vi "Facade Line Chart.vi"(0 "Data In":T4, 2 "Display State In":T2, 3 "Container State":T3) -> (6 "Data Out":T4, 7 "Display State Out":T2, 8 "Action":T1)   [LabVIEW 2016, in "Line Chart.xctl"]
uses:
  Line Chart.xctl
  Data Line Chart.ctl
  <vilib>/_xctls/Container State.ctl
  State Line Chart.ctl
  <vilib>/_xctls/Action.ctl
  <vilib>/_xctls/XControlSupport.lvlib
panel:
  in  "ActiveX Container":refnum<k7>(container)
types:
  T1 = typedef "XControlSupport.lvlib/Action.ctl" = cluster{"Data Changed?":bool, "State Changed?":bool, "Action Name":string}
  T2 = typedef "Line Chart.xctl/State Line Chart.ctl" = cluster{"Numeric":dbl}
  T3 = typedef "XControlSupport.lvlib/Container State.ctl" = cluster{"Indicator?":bool, "Run Mode?":bool, " Refnum":refnum<vi>}
  T4 = typedef "Line Chart.xctl/Data Line Chart.ctl" = cluster{"X-Axis":string[], "Plots":cluster{"Data":dbl[], "Label":string, "Y-Axis":enum16{"Y-Axis 1", "Y-Axis 2"}, "Color":u32}[], "Plot Title":string}
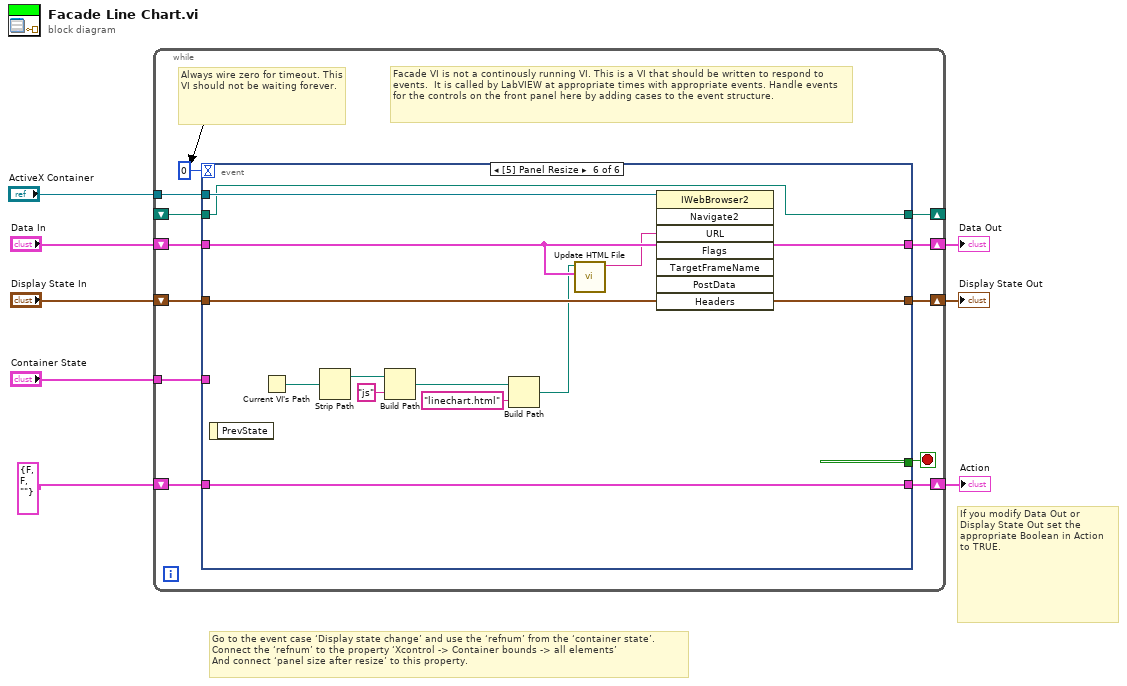
[diagram p0: block diagram]
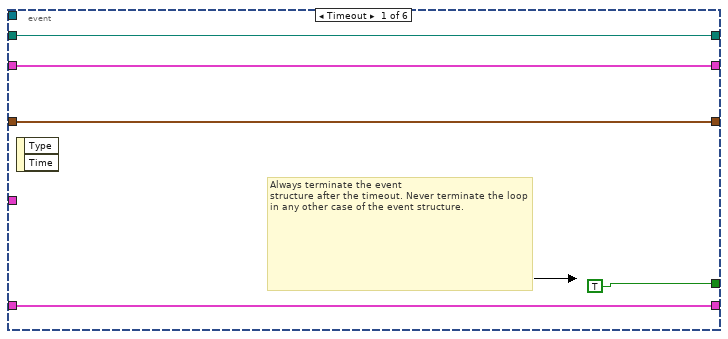
[diagram p2: hidden frame]
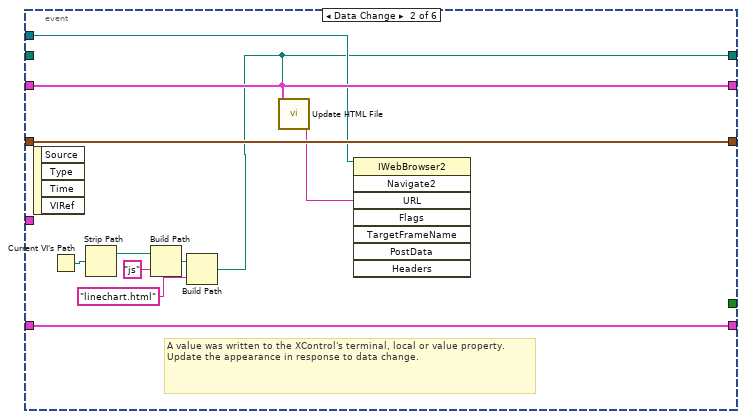
[diagram p3: hidden frame]
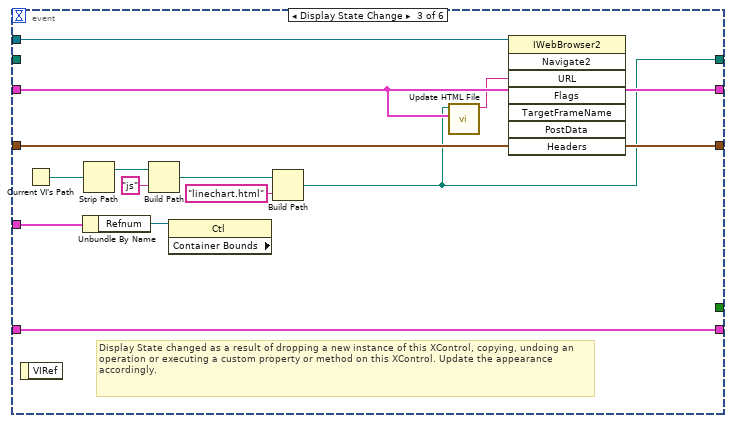
[diagram p4: hidden frame]
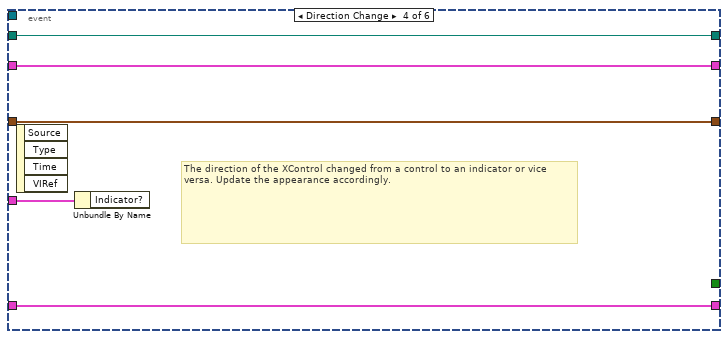
[diagram p5: hidden frame]
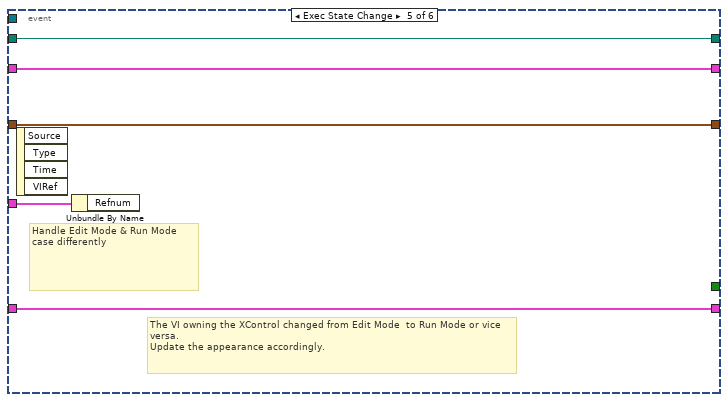
[diagram p6: hidden frame]
diagram:
  # "Go to the event case ‘Display state change’ and use the ‘refnum’ from the ‘container state’.\nConnect the ‘refnum’ to the property ‘Xcontrol -> Container bounds -> all elements’\nAnd connect ‘panel size after resize’ to this property."
  # "If you modify Data Out or\nDisplay State Out set the\nappropriate Boolean in Action\nto TRUE."
  n1 = while {
    shift-right: [w19] -> w5
    shift-left: "Display State In" -> [w20]
    tunnel: "Container State" -> [w16]
    shift-right: [w14] -> w8
    shift-left: "Data In" -> [w15]
    shift-right: [w12] -> w3
    shift-left: T1 {"Data Changed?"=FALSE, "State Changed?"=FALSE, "Action Name"=""} ("Action") -> [w13]
    tunnel: "ActiveX Container" -> [w11]
    shift-right: [w10] -> _
    shift-left: _ -> [w9]
    stop <- w18 stop-if-true
    # "Facade VI is not a continously running VI. This is a VI that should be written to respond to events.  It is called by LabVIEW at appropriate times with appropriate events. Handle events for the controls on the front panel here by adding cases to the event structure."
    # "Always wire zero for timeout. This\nVI should not be waiting forever."
    n2 = event shown="[5] Panel Resize" {
      selector: _ -> [_ _ _ _ _ _]
      dyn-events: _ -> [_ _ _ _ _ _]
      timeout: 0 -> [_ _ _ _ _ _]
      tunnel: w20 -> [w23 w36 w49 w53 w58 w71]
      tunnel: [w23 w36 w49 w53 w58 w71] -> w19
      tunnel: [TRUE _ _ _ _ _] -> w18
      tunnel: w16 -> [_ _ w47 w54 w59 _]
      tunnel: w15 -> [w22 w34 w39 w52 w57 w68]
      tunnel: [w22 w34 w39 w52 w57 w68] -> w14
      tunnel: [w24 w35 w48 w51 w56 w70] -> w12
      tunnel: w13 -> [w24 w35 w48 w51 w56 w70]
      tunnel: w11 -> [_ w33 w41 _ _ w69]
      tunnel: [w21 w31 w38 w50 w55 w67] -> w10
      tunnel: w9 -> [w21 _ _ w50 w55 w67]
      event Timeout {
        # "Always terminate the event\nstructure after the timeout. Never terminate the loop in any other case of the event structure."
        n3 = event-data() -> ()  [unwired: 1 in, 2 out]
      }
      event Data Change {
        # "A value was written to the XControl's terminal, local or value property.\nUpdate the appearance in response to data change."
        n4 = event-data() -> ()  [unwired: 1 in, 4 out]
        n5 = Current VI's Path() -> (path=w30:path)
        n6 = Strip Path(path=w30) -> (stripped path=w29:path)  [unwired: 1 out]
        n7 = Build Path(base path=w29, name or relative path="js") -> (appended path=w27:path)
        n8 = Build Path(base path=w27, name or relative path="linechart.html") -> (appended path=w31:path)
        n9 = call "Update HTML File.vi"("Data In"=w34, "Path"=w31) -> ("URL out"=w32:string)  [unwired: 9 in]
        n10 = invoke class="IWebBrowser2" method="Navigate2"(reference=w33, "URL"=w32) -> ()  [unwired: 6 in, 8 out]
      }
      event Display State Change {
        # "Display State changed as a result of dropping a new instance of this XControl, copying, undoing an operation or executing a custom property or method on this XControl. Update the appearance accordingly."
        n11 = event-data() -> ()  [unwired: 1 in, 1 out]
        n12 = Current VI's Path() -> (path=w46:path)
        n13 = Unbundle By Name(w47) -> ("Refnum"=w40:refnum<vi>)
        n14 = Strip Path(path=w46) -> (stripped path=w45:path)  [unwired: 1 out]
        n15 = Build Path(base path=w45, name or relative path="js") -> (appended path=w43:path)
        n16 = property class="Ctl" props=["Container Bounds"](reference=w40) -> ()  [unwired: 1 in, 3 out]
        n17 = Build Path(base path=w43, name or relative path="linechart.html") -> (appended path=w38:path)
        n18 = call "Update HTML File.vi"("Data In"=w39, "Path"=w38) -> ("URL out"=w37:string)  [unwired: 9 in]
        n19 = invoke class="IWebBrowser2" method="Navigate2"(reference=w41, "URL"=w37) -> ()  [unwired: 6 in, 8 out]
      }
      event Direction Change {
        # "The direction of the XControl changed from a control to an indicator or vice versa. Update the appearance accordingly."
        n20 = event-data() -> ()  [unwired: 1 in, 4 out]
        n21 = Unbundle By Name(w54) -> ()  [unwired: 1 out]
      }
      event Exec State Change {
        # "The VI owning the XControl changed from Edit Mode  to Run Mode or vice versa.\nUpdate the appearance accordingly."
        # "Handle Edit Mode & Run Mode\ncase differently"
        n22 = event-data() -> ()  [unwired: 1 in, 4 out]
        n23 = Unbundle By Name(w59) -> ()  [unwired: 1 out]
      }
      event Panel Resize {
        n24 = event-data() -> ()  [unwired: 1 in, 1 out]
        n25 = Current VI's Path() -> (path=w65:path)
        n26 = Strip Path(path=w65) -> (stripped path=w64:path)  [unwired: 1 out]
        n27 = Build Path(base path=w64, name or relative path="js") -> (appended path=w62:path)
        n28 = Build Path(base path=w62, name or relative path="linechart.html") -> (appended path=w60:path)
        n29 = call "Update HTML File.vi"("Data In"=w68, "Path"=w60) -> ("URL out"=w66:string)  [unwired: 9 in]
        n30 = invoke class="IWebBrowser2" method="Navigate2"(reference=w69, "URL"=w66) -> ()  [unwired: 6 in, 8 out]
      }
    }
  }
  "Display State Out" <- w5
  "Data Out" <- w8
  "Action" <- w3
